vi "detector_get_counts_1d_dbl.vi"(8 "error in (no error)":errorcluster, 11 "lightfield_class in":refnum<class "lightfield_class.lvclass">) -> (0 "error out":errorcluster, 2 "counts":dbl[](array[numeric]), 3 "lightfield_class out":refnum<class "lightfield_class.lvclass">)   [LabVIEW 2015, in "lightfield_class.lvclass"]
uses:
  lightfield_class.lvclass
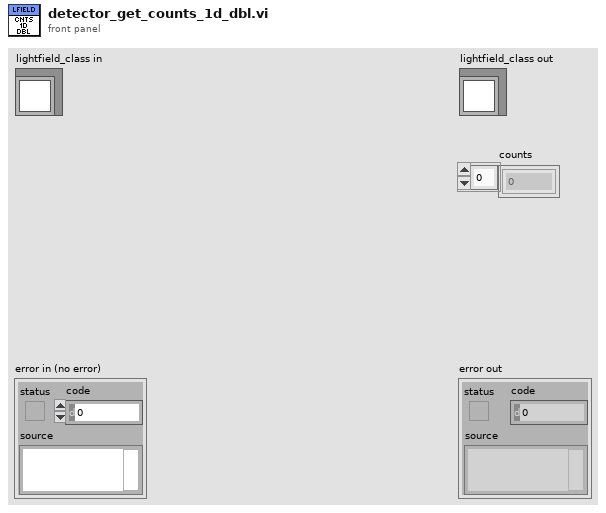
[diagram p1: front panel]
types:
  T1 = cluster{"Image":dbl[][][], "Frame Size":cluster{"F":i32, "Y":i32, "X":i32}}
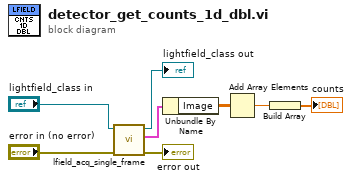
[diagram p0: block diagram]
diagram:
  n1 = call "lfield_acq_single_frame.vi"("error in (no error)"="error in (no error)", "lightfield_class in"="lightfield_class in") -> ("error out"=→"error out":errorcluster, "image_data"=w5:T1, "lightfield_class out"=→"lightfield_class out":refnum<class "lightfield_class.lvclass">)  [unwired: 7 in]
  n2 = Unbundle By Name(w5) -> ("Image"=w4:dbl[][][])
  n3 = Add Array Elements(numeric array=w4) -> (sum=w3:dbl)
  n4 = Build Array(w3) -> (→"counts":dbl[])
